vi "TIFF-Append Tag (U16 1D).vi"(0 "IFD in":u8[](array[numeric]), 5 "[IN] TagID":u16, 7 "[IN] DataType":u16(ring)=4 items=["BYTE"=1, "ASCII"=2, "SHORT"=3, "LONG"=4, "RATIONAL"=5], 9 "[IN] Data":u16[](array[numeric]), 11 "error IN":errorcluster, 12 "[IN] Byte order":T1(ring)) -> (4 "IFD out":u8[](array[numeric]), 15 "error OUT":errorcluster)   [LabVIEW 2020]
doc: "This VI writes a tif TAG. Input data is an array of U32. Note that the data should not be larger than 4 bytes."
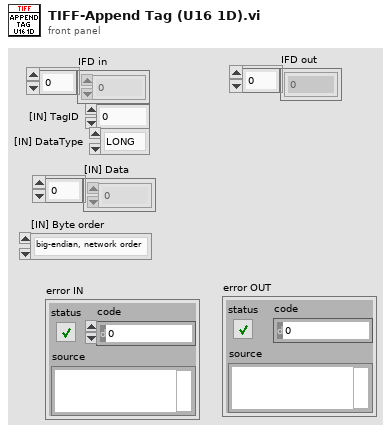
[diagram p1: front panel]
types:
  T1 = enum16{"big-endian, network order", "native, host order", "little-endian"}
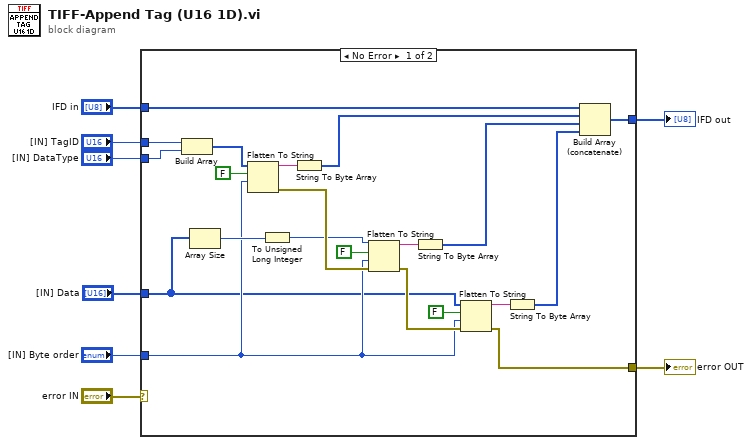
[diagram p0: block diagram]
diagram:
  n1 = case shown="No Error" "error IN" {
    selector: "error IN" -> [_ w31]
    tunnel: [w12 w31] -> w8
    tunnel: "[IN] Byte order" -> [w11 _]
    tunnel: "[IN] Data" -> [w10 _]
    tunnel: "[IN] TagID" -> [w29 _]
    tunnel: "[IN] DataType" -> [w28 _]
    tunnel: "IFD in" -> [w22 w30]
    tunnel: [w19 w30] -> w1
    frame No Error {
      n2 = Build Array(w29, w28) -> (w25:u16[])
      n3 = Array Size(array=w10) -> (size(s)=w16:i32)
      n4 = Flatten To String(anything=w25, prepend array or string size? (T)=FALSE, byte order (0:big-endian, network order)=w11) -> (data string=w27:string, error out=w18:errorcluster)  [unwired: 1 in, 1 out]
      n5 = To Unsigned Long Integer(number=w16) -> (unsigned 32bit integer=w17:u32)
      n6 = String To Byte Array(string=w27) -> (unsigned byte array=w21:u8[])
      n7 = Flatten To String(anything=w17, prepend array or string size? (T)=FALSE, byte order (0:big-endian, network order)=w11, error in (no error)=w18) -> (data string=w24:string, error out=w13:errorcluster)  [unwired: 1 out]
      n8 = String To Byte Array(string=w24) -> (unsigned byte array=w20:u8[])
      n9 = Flatten To String(anything=w10, prepend array or string size? (T)=FALSE, byte order (0:big-endian, network order)=w11, error in (no error)=w13) -> (data string=w15:string, error out=w12:errorcluster)  [unwired: 1 out]
      n10 = String To Byte Array(string=w15) -> (unsigned byte array=w9:u8[])
      n11 = Build Array (concatenate)(w22, w21, w20, w9) -> (w19:u8[])
    }
    frame Error {
    }
  }
  "error OUT" <- w8
  "IFD out" <- w1
